vi "Move to Wavelength (TRIAX).vi"(7 "Mono System # (0)":T1, 8 "error in (no error)":errorcluster, 10 "Target wavelength":dbl[unit], 11 "VISA resource name":refnum<visa-resource-name>) -> (0 "error out":errorcluster, 3 "VISA resource name out":refnum<visa-resource-name>)   [LabVIEW 2023, in "JY-SPEX-TRIAX.lvlib"]
doc: "Moves the spectrometer's grating to a specific wavelength according to the base grating (1200 grooves/mm).\n\n<B>Note: only works with TRIAX series monochromators.</B>"
uses:
  JY-SPEX-TRIAX.lvlib
  controls.llb/Monochromator System Number.ctl
  Spectrometer Config.vi
panel:
  out "Backlash":dbl[unit]
  out "Distance":dbl[unit]
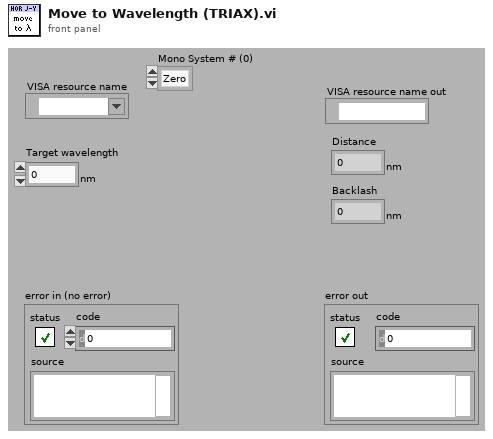
[diagram p1: front panel]
types:
  T1 = typedef "JY-SPEX-TRIAX.lvlib/Monochromator System Number.ctl" = enum16{"Zero", "One"}
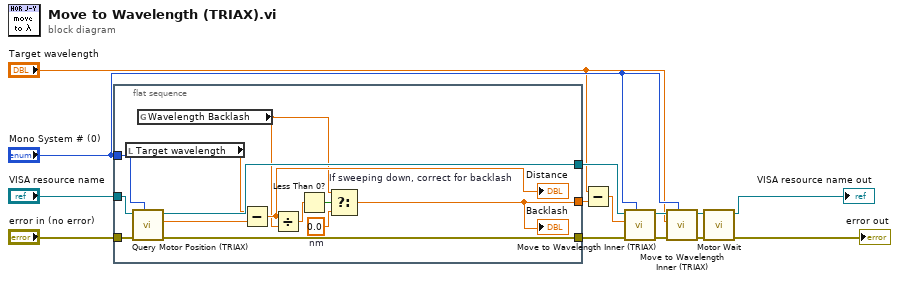
[diagram p0: block diagram]
diagram:
  n1 = flat-sequence {
    tunnel: "VISA resource name" -> [w27]
    tunnel: [w26] -> w12
    tunnel: "error in (no error)" -> [w25]
    tunnel: [w24] -> w10
    tunnel: "Mono System # (0)" -> [w21]
    tunnel: [w15] -> w5
    frame #0 {
      w16 = dbl[unit] 0.0  # nm
      n2 = local read "Target wavelength"() -> (w23:dbl[unit])
      n3 = call "Query Motor Position (TRIAX).vi"("Mono System # (0)"=w21, "error in (no error)"=w25, "VISA resource name"=w27) -> ("error out"=w24:errorcluster, "wavelength"=w22:dbl[unit], "VISA resource name out"=w26:refnum<visa-resource-name>)  [unwired: 6 out]
      n4 = global read "Spectrometer Config.vi" "Wavelength Backlash"() -> (w17:dbl[unit])
      n5 = Subtract(x=w23, y=w22) -> (x-y=w18:dbl[unit])
      "Distance" <- w18
      n6 = Divide(x=w18, y=w17) -> (x/y=w19:dbl)
      n7 = Less Than 0?(x=w19) -> (x < 0?=w20:bool)
      n8 = Select "If sweeping down, correct for backlash"(t=w17, s=w20, f=w16) -> (s? t:f=w15:dbl[unit])
      "Backlash" <- w15
    }
  }
  n9 = Subtract(x="Target wavelength", y=w5) -> (x-y=w7:dbl[unit])
  n10 = call "Move to Wavelength Inner (TRIAX).vi"("Mono System # (0)"="Mono System # (0)", "error in (no error)"=w10, "wavelength"=w7, "VISA resource name"=w12) -> ("error out"=w9:errorcluster, "VISA resource name out"=w13:refnum<visa-resource-name>)  [unwired: 6 out]
  n11 = call "Move to Wavelength Inner (TRIAX).vi"("Mono System # (0)"="Mono System # (0)", "error in (no error)"=w9, "wavelength"="Target wavelength", "VISA resource name"=w13) -> ("error out"=w2:errorcluster, "VISA resource name out"=w4:refnum<visa-resource-name>)  [unwired: 6 out]
  n12 = call "Motor Wait.vi"("error in"=w2, "VISA resource name in"=w4) -> ("error out"=→"error out":errorcluster, "VISA resource name out"=→"VISA resource name out":refnum<visa-resource-name>)  [unwired: 8 out]
